vi "Config-Identity.vi"(8 "error in":errorcluster, 11 "Refnum in":T3) -> (0 "error out":errorcluster, 2 "Identity":T1={"NodeID"="", "Role"=enum."Sender"}, 3 "Refnum out":T3)   [LabVIEW 2021, in "UDP_Config.lvclass"]
uses:
  UDP_Config.lvclass
  <vilib>/Utility/config.llb/Config Data RefNum.ctl
  Control/Identity.ctl
  Control/Role.ctl
  <vilib>/Utility/config.llb/Read Key (String).vi
  <vilib>/Utility/config.llb/NI_LVConfig.lvlib
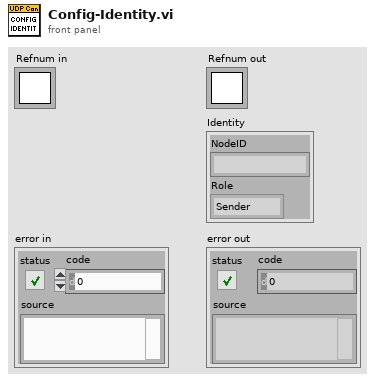
[diagram p1: front panel]
types:
  T1 = typedef "Identity.ctl" = cluster{"NodeID":string, "Role":T2}
  T2 = typedef "Role.ctl" = enum16{"Undefined", "Sender", "Receiver"}
  T3 = typedef "NI_LVConfig.lvlib/Config Data RefNum.ctl" = refnum<k1>
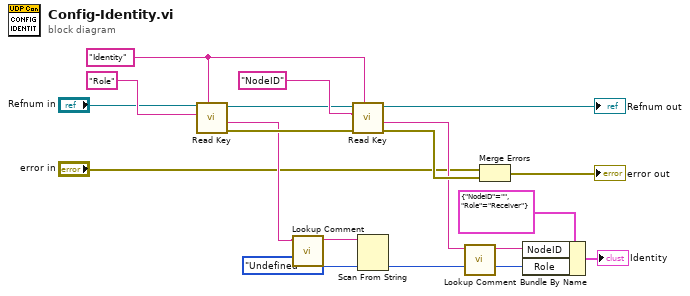
[diagram p0: block diagram]
diagram:
  w14 = "Identity" ("key")
  n1 = call-poly <vilib>:"Read Key.vi"("section"=w14, "key"="Role", "refnum"="Refnum in") -> ("error out"=w16:errorcluster, "value"=w6:string, "refnum out"=w13:T3)  [unwired: 5 in, 1 out]
  n2 = call "Lookup Comment.vi"("String in"=w6) -> ("Value"=w5:string)  [unwired: 3 in, 1 out]
  n3 = call-poly <vilib>:"Read Key.vi"("section"=w14, "error in (no error)"=w16, "key"="NodeID", "refnum"=w13) -> ("error out"=w17:errorcluster, "value"=w3:string, "refnum out"=→"Refnum out":T3)  [unwired: 4 in, 1 out]
  n4 = Scan From String(input string=w5, default 1=Role."Undefined" ("Role")) -> (output 1=w8:T2)  [unwired: 3 in, 3 out]
  n5 = call "Lookup Comment.vi"("String in"=w3) -> ("Value"=w4:string)  [unwired: 3 in, 1 out]
  n6 = Merge Errors("error in", w17) -> (→"error out":errorcluster)
  n7 = Bundle By Name(cluster=T1 {"NodeID"="", "Role"=enum."Receiver"} ("Identity"), "NodeID"=w4, "Role"=w8) -> (→"Identity":T1)
